vi "Rx Message to Transfer Handle.vi"(8 "error in":errorcluster, 9 "message":T2={"name"="", "message type"="BC to RT", "endpoint Tx"={"terminal address"=0, "subaddress"=0}, "endpoint Rx"={"terminal address"=0, "subaddress"=0}, "create timestamp channel"=FALSE, "mode code"=0, "number of words"=0, "parameters"=[]}, 10 "remote terminal handles":u64[](array[numeric]), 11 "bus controller handle":u64) -> (0 "error out":errorcluster, 3 "Rx read info":T1)   [LabVIEW 2020, in "Ballard MIL-STD-1553 Engine.lvlib" / "Custom Device.lvlib"]
uses:
  Custom Device.lvlib
  Shared/Message Definition.ctl
  Shared/Message Type.ctl
  Shared/Terminal Endpoint.ctl
  Shared/Address.ctl
  Shared/Parameter Definition.ctl
  Shared/Rx Read Info.ctl
  <instrlib>/BTI1553Lib/Public/Controls/1553 RT Transfer Type.ctl
  <instrlib>/BTI1553Lib/Public/Controls/1553 Transfer Direction.ctl
  <instrlib>/BTI1553Lib/Private/RT/Configure/Get RT Xfer Handle.vi
  <instrlib>/BTI1553Lib/BTI1553LV.lvlib
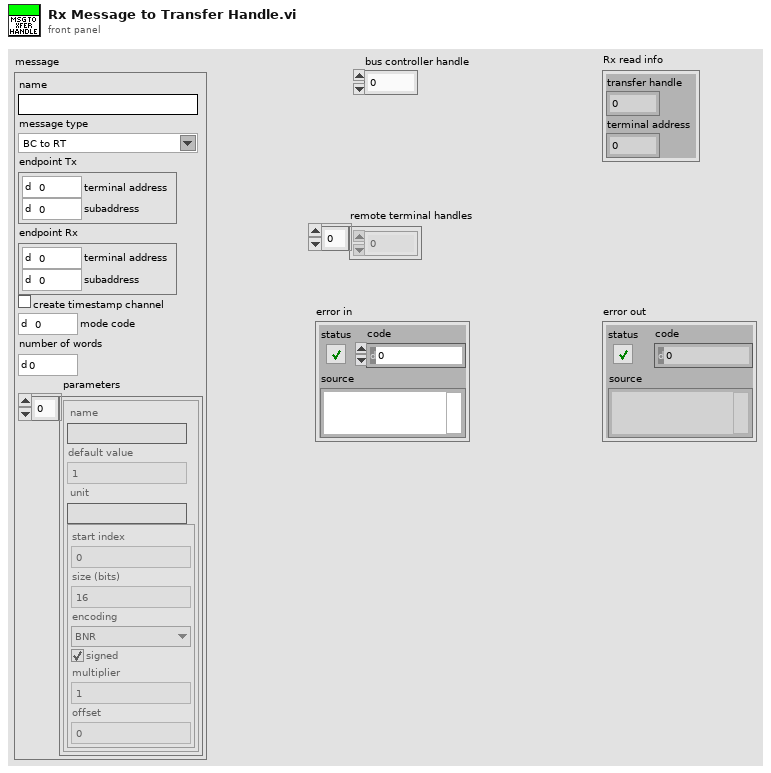
[diagram p1: front panel]
types:
  T1 = typedef "Rx Read Info.ctl" = cluster{"transfer handle":u64, "terminal address":u16}
  T2 = typedef "Message Definition.ctl" = cluster{"name":string, "message type":T3, "endpoint Tx":T4, "endpoint Rx":T4, "create timestamp channel":bool, "mode code":u16, "number of words":u16, "parameters":cluster{"name":string, "default value":dbl, "unit":string, "parameter definition":T6}[]}
  T3 = typedef "Message Type.ctl" = string
  T4 = typedef "Terminal Endpoint.ctl" = cluster{"terminal address":T5, "subaddress":T5}
  T5 = typedef "Address.ctl" = u16
  T6 = typedef "Parameter Definition.ctl" = cluster{"start index":i32, "size (bits)":i32, "encoding":enum16{"BNR", "BCD", "Discrete"}, "signed":bool, "multiplier":dbl, "offset":dbl}
  T7 = typedef "BTI1553LV.lvlib/1553 Transfer Direction.ctl" = u32
  T8 = typedef "BTI1553LV.lvlib/1553 RT Transfer Type.ctl" = u32
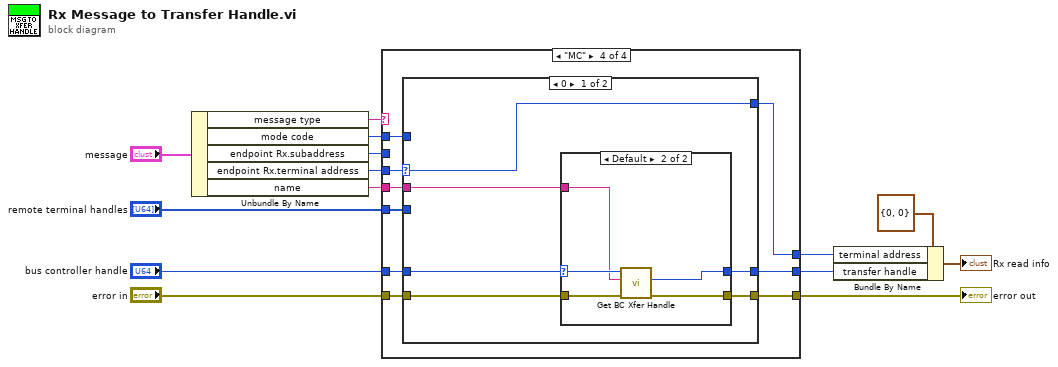
[diagram p0: block diagram]
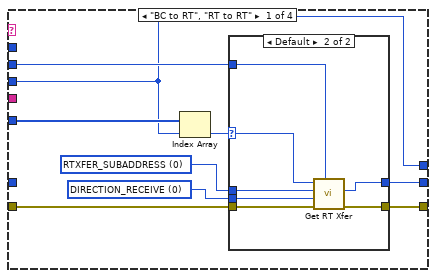
[diagram p2: hidden frame]
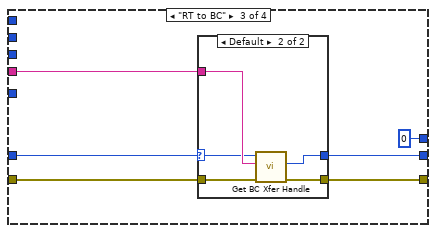
[diagram p5: hidden frame]
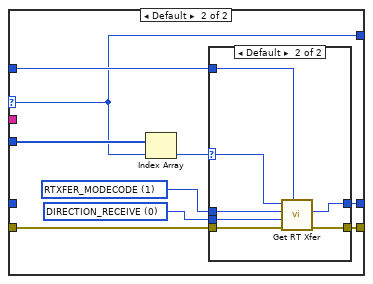
[diagram p8: hidden frame]
diagram:
  n1 = Unbundle By Name("message") -> ("message type"=w5:T3, "mode code"=w11:u16, "endpoint Rx.subaddress"=w14:T5, "endpoint Rx.terminal address"=w13:T5, "name"=w6:string)
  n2 = case shown="\"MC\"" w5 {
    tunnel: w14 -> [w16 _ _ _]
    tunnel: w13 -> [w15 _ _ w53]
    tunnel: w11 -> [_ _ _ w49]
    tunnel: "error in" -> [w23 w32 w36 w52]
    tunnel: "remote terminal handles" -> [w20 _ _ w50]
    tunnel: [w18 _ w38 w48] -> w1
    tunnel: [w17 w32 w35 w51] -> w8
    tunnel: "bus controller handle" -> [_ _ w37 w47]
    tunnel: w6 -> [_ _ w33 w46]
    tunnel: [w15 _ T5 0 ("terminal address") w45] -> w2
    frame "BC to RT", "RT to RT" {
      w22 = T7 0 items=["DIRECTION_RECEIVE", "DIRECTION_TRANSMIT"] ("transfer direction")
      w21 = T8 0 items=["RTXFER_SUBADDRESS", "RTXFER_MODECODE"] ("transfer type")
      n3 = Index Array(array=w20, index=w15) -> (element=w19:u64)
      n4 = case shown="Default" w19 {
        selector: w19 -> [_ w28]
        tunnel: w23 -> [w24 w31]
        tunnel: w22 -> [_ w30]
        tunnel: w21 -> [_ w29]
        tunnel: [_ w27] -> w18
        tunnel: [w24 w26] -> w17
        tunnel: w16 -> [_ w25]
        frame 0, -1 {
        }
        frame Default {
          n5 = call-poly <instrlib>:"Get RT Xfer.vi"("transfer sa number or mc number"=w25, "error in (no error)"=w31, "transfer direction"=w30, "transfer type"=w29, "remote terminal handle in"=w28) -> ("error out"=w26:errorcluster, "rt transfer handle out"=w27:u64)  [unwired: 4 in, 1 out]
        }
      }
    }
    frame Default {
    }
    frame "RT to BC" {
      n6 = case shown="Default" w37 {
        selector: w37 -> [_ w42]
        tunnel: [_ w44] -> w38
        tunnel: w33 -> [_ w43]
        tunnel: w36 -> [w39 w41]
        tunnel: [w39 w40] -> w35
        frame 0, -1 {
        }
        frame Default {
          n7 = call <instrlib>:"Get BC Xfer Handle.vi"("error in (no error)"=w41, "bc transfer name"=w43, "bus controller handle in"=w42) -> ("error out"=w40:errorcluster, "bc transfer handle out"=w44:u64)  [unwired: 6 in, 1 out]
        }
      }
    }
    frame "MC" {
      n8 = case shown="0" w53 {
        selector: w53 -> [w55 w66]
        tunnel: w52 -> [w59 w74]
        tunnel: [w58 w73] -> w51
        tunnel: w50 -> [_ w70]
        tunnel: w49 -> [_ w68]
        tunnel: [w56 w67] -> w48
        tunnel: w47 -> [w57 _]
        tunnel: w46 -> [w54 _]
        tunnel: [w55 w66] -> w45
        frame 0 {
          n9 = case shown="Default" w57 {
            selector: w57 -> [_ w63]
            tunnel: w59 -> [w60 w65]
            tunnel: [w60 w64] -> w58
            tunnel: w54 -> [_ w62]
            tunnel: [_ w61] -> w56
            frame 0, -1 {
            }
            frame Default {
              n10 = call <instrlib>:"Get BC Xfer Handle.vi"("error in (no error)"=w65, "bc transfer name"=w62, "bus controller handle in"=w63) -> ("error out"=w64:errorcluster, "bc transfer handle out"=w61:u64)  [unwired: 6 in, 1 out]
            }
          }
        }
        frame Default {
          w71 = T8 1 items=["RTXFER_SUBADDRESS", "RTXFER_MODECODE"] ("transfer type")
          w72 = T7 0 items=["DIRECTION_RECEIVE", "DIRECTION_TRANSMIT"] ("transfer direction")
          n11 = Index Array(array=w70, index=w66) -> (element=w69:u64)
          n12 = case shown="Default" w69 {
            selector: w69 -> [_ w78]
            tunnel: w74 -> [w75 w82]
            tunnel: [w75 w81] -> w73
            tunnel: w72 -> [_ w80]
            tunnel: w71 -> [_ w79]
            tunnel: w68 -> [_ w77]
            tunnel: [_ w76] -> w67
            frame 0, -1 {
            }
            frame Default {
              n13 = call-poly <instrlib>:"Get RT Xfer.vi"("transfer sa number or mc number"=w77, "error in (no error)"=w82, "transfer direction"=w80, "transfer type"=w79, "remote terminal handle in"=w78) -> ("error out"=w81:errorcluster, "rt transfer handle out"=w76:u64)  [unwired: 4 in, 1 out]
            }
          }
        }
      }
    }
  }
  "error out" <- w8
  n14 = Bundle By Name(cluster=T1 {"transfer handle"=0, "terminal address"=0} ("Rx read info"), "terminal address"=w2, "transfer handle"=w1) -> (→"Rx read info":T1)
